vi "Echo_Record.vi"(10 "Record":bool, 11 "file name":path) -> ()   [LabVIEW 2012]
uses:
  Echo_Global_Data.vi
  <vilib>/Utility/file.llb/Write To Spreadsheet File (DBL).vi
panel:
  # "This VI is contained in Echo Periodic Tasks\n\nIt does not need to be placed anywhere.\n\nIt takes the global variables:\n -Echo Recorded Data 01 through\n -Echo Recorded Data 10\nAnd uses Echo Record Values to generate\na 2D array.\n\nIt takes this data from Echo Record\nValues and converts them to a\nformat of 250 x 11.  Each row represents\na time linearly spaced between the\nminimum and maximum times.\n\nIt then writes them to a spreadsheet."
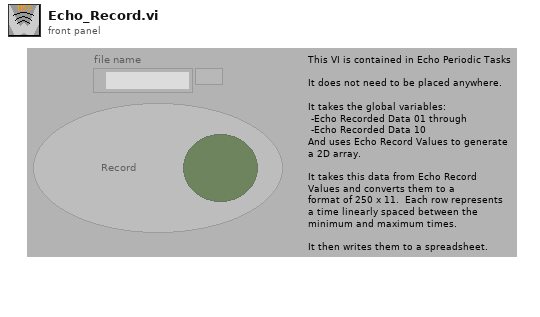
[diagram p1: front panel]
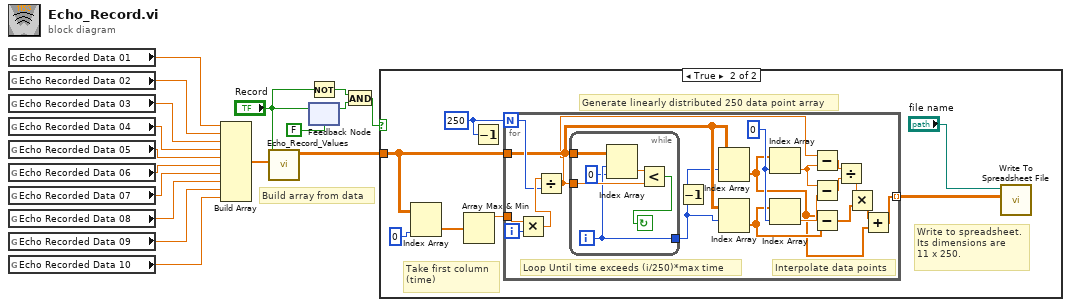
[diagram p0: block diagram]
diagram:
  # "Build array from data"
  n1 = global read "Echo_Global_Data.vi" "Echo Recorded Data 01"() -> (w11:dbl)
  n2 = global read "Echo_Global_Data.vi" "Echo Recorded Data 02"() -> (w10:dbl)
  n3 = global read "Echo_Global_Data.vi" "Echo Recorded Data 03"() -> (w9:dbl)
  n4 = global read "Echo_Global_Data.vi" "Echo Recorded Data 04"() -> (w8:dbl)
  n5 = global read "Echo_Global_Data.vi" "Echo Recorded Data 05"() -> (w7:dbl)
  n6 = global read "Echo_Global_Data.vi" "Echo Recorded Data 06"() -> (w6:dbl)
  n7 = global read "Echo_Global_Data.vi" "Echo Recorded Data 07"() -> (w5:dbl)
  n8 = global read "Echo_Global_Data.vi" "Echo Recorded Data 08"() -> (w4:dbl)
  n9 = global read "Echo_Global_Data.vi" "Echo Recorded Data 09"() -> (w3:dbl)
  n10 = global read "Echo_Global_Data.vi" "Echo Recorded Data 10"() -> (w2:dbl)
  n11 = Build Array(w11, w10, w9, w8, w7, w6, w5, w4, w3, w2) -> (w1:dbl[])
  n12 = call "Echo_Record_Values.vi"("Data"=w1, "Record"="Record") -> ("Out"=w17:dbl[][])  [unwired: 9 out]
  n13 = Not(x="Record") -> (.not. x?=w15:bool)
  n14 = feedback-in #1("Record") -> ()
  n15 = feedback #1(FALSE ("Button 1")) -> (w13:bool)
  n16 = And(x=w15, y=w13) -> (x .and. y?=w16:bool)
  n17 = case shown="True" w16 {
    tunnel: w17 -> [_ w24]
    frame False {
      # "Do nothing except on the loop that the button turns false\nExample:\n\n         button value for           button value for\n           current loop                        previous loop                                         result\n\n                false                                    false                                                  false\n                false                                    true                                                   true\n                true                                     false                                                  false\n                true                                     true                                                   false"
    }
    frame True {
      w22 = 250
      # "Write to spreadsheet.\nIts dimensions are\n11 x 250."
      # "Take first column\n(time)"
      # "Generate linearly distributed 250 data point array"
      n18 = Index Array(array=w24, index (col)=0 ("index (row)")) -> (element=w23:dbl[])  [unwired: 1 in]
      n19 = Array Max & Min(array=w23) -> (max value=w21:dbl)  [unwired: 3 out]
      n20 = Decrement(x=w22) -> ()  [unwired: 1 out]
      n21 = for {
        N: w22 -> [w40]
        tunnel: w24 -> [w39]
        tunnel: w21 -> [w43]
        tunnel: [w29] -> w20 mode=indexing
        i -> [w42]
        w38 = 0
        # "Interpolate data points"
        # "Loop Until time exceeds (i/250)*max time"
        n22 = Multiply(x=w43, y=w42) -> (x*y=w41:dbl)
        n23 = Divide(x=w41, y=w40) -> (x/y=w26:dbl)
        n24 = while {
          tunnel: w26 -> [w49]
          tunnel: w39 -> [w48]
          tunnel: [w45] -> w27
          i -> [w45]
          stop <- w46 continue-if-true
          n25 = Index Array(array=w48, index (row)=w45, index (col)=0 ("disabled index (col)")) -> (element=w47:dbl)
          n26 = Less?(x=w47, y=w49) -> (x < y?=w46:bool)
        }
        n27 = Decrement(x=w27) -> (x-1=w28:i32)
        n28 = Index Array(array=w39, index (row)=w28) -> (element=w30:dbl[])  [unwired: 1 in]
        n29 = Index Array(array=w39, index (row)=w27) -> (element=w34:dbl[])  [unwired: 1 in]
        n30 = Index Array(array=w30, index=w38) -> (element=w37:dbl)
        n31 = Index Array(array=w34, index=w38) -> (element=w32:dbl)
        n32 = Subtract(x=w26, y=w37) -> (x-y=w35:dbl)
        n33 = Subtract(x=w37, y=w32) -> (x-y=w36:dbl)
        n34 = Subtract(x=w30, y=w34) -> (x-y=w33:dbl[])
        n35 = Divide(x=w35, y=w36) -> (x/y=w25:dbl)
        n36 = Multiply(x=w25, y=w33) -> (x*y=w31:dbl[])
        n37 = Add(x=w31, y=w30) -> (x+y=w29:dbl[])
      }
      n38 = call-poly <vilib>:"Write To Spreadsheet File.vi"("2D data"=w20, "file path (dialog if empty)"="file name") -> ()  [unwired: 4 in, 3 out]
    }
  }
